vi "Run.vi"(7 "Team Index":i32, 8 "Column":i32, 9 "Row":i32, 10 "View":i32[](array[numeric]) caption="View (Team Index, -1: empty)", 11 "Test In":refnum<class "Swarm.lvclass">) -> (0 "Replicated":refnum<class "Square.lvclass">, 1 "Direction":T1, 2 "Action":T2, 3 "Square Out":refnum<class "Square.lvclass">)   [LabVIEW 2017, in "Swarm.lvclass"]
uses:
  Swarm.lvclass
  C:/Workspace/Endigit/SquareBattle/Square/Square.lvclass
  Square/Square.lvclass
  Type Defs/Action Enum.ctl
  Type Defs/Direction Enum.ctl
  Common/Position.ctl
  Swarm.lvclass/Swarm.ctl
  SubVIs/Read-Only Globals.vi
  SubVIs/Globals (private).vi
  Common/Common.lvlib
  Type Defs/SB Type Defs.lvlib
panel:
  # "NW\nN\nNE\nE\nSE\nS\nSW\nW"
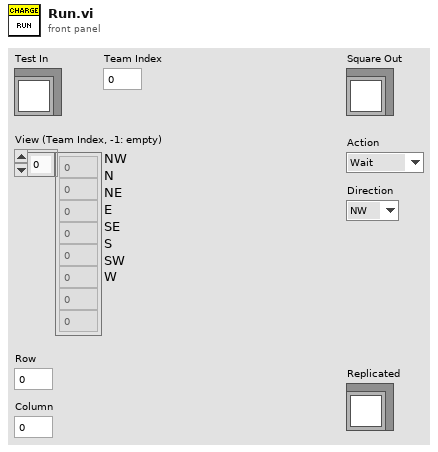
[diagram p1: front panel]
types:
  T1 = typedef "SB Type Defs.lvlib/Direction Enum.ctl" = enum16{"NW", "N", "NE", "E", "SE", "S", "SW", "W"}
  T2 = typedef "SB Type Defs.lvlib/Action Enum.ctl" = enum16{"Wait", "Move", "Attack", "Replicate"}
  T3 = typedef "Common.lvlib/Position.ctl" = cluster{"Column":i32, "Row":i32}
  T4 = typedef "Common.lvlib/Map DVR.ctl" = refnum<data-value>
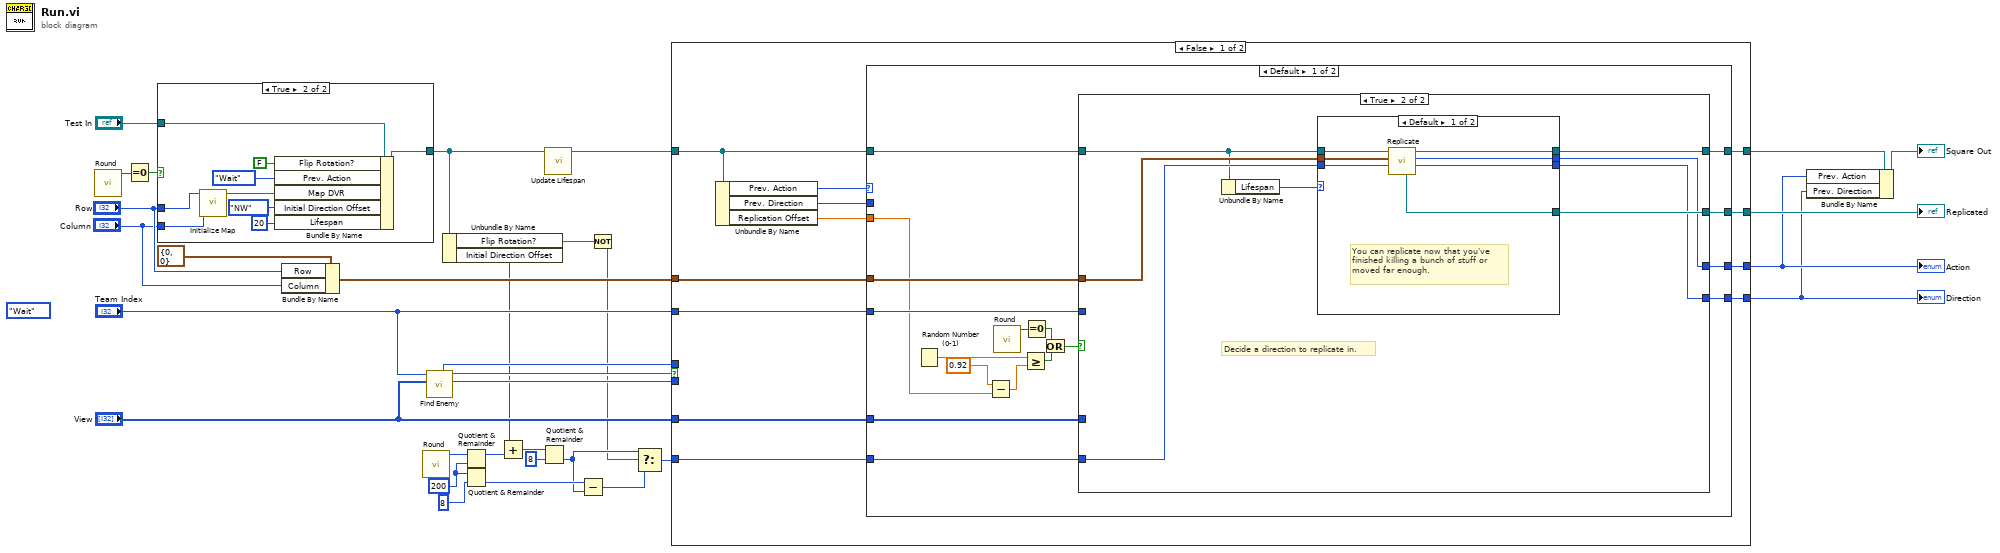
[diagram p0: block diagram]
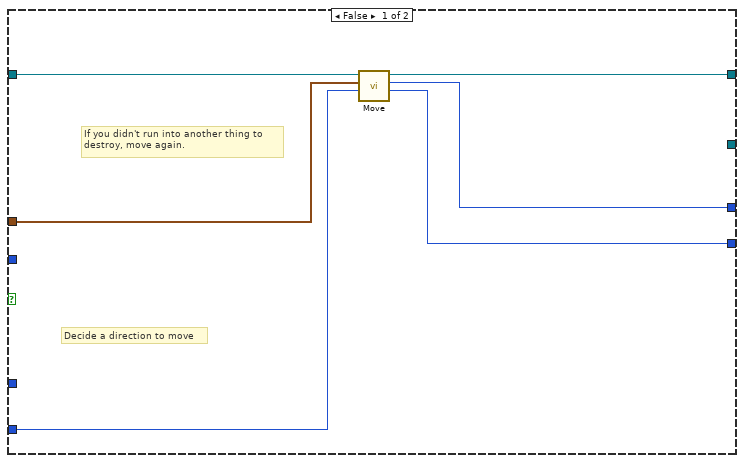
[diagram p3: hidden frame]
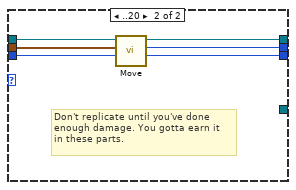
[diagram p4: hidden frame]
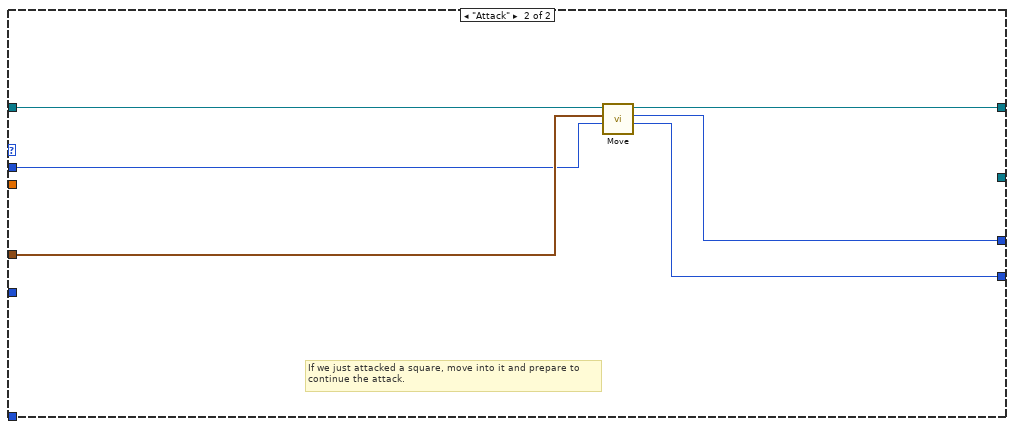
[diagram p5: hidden frame]
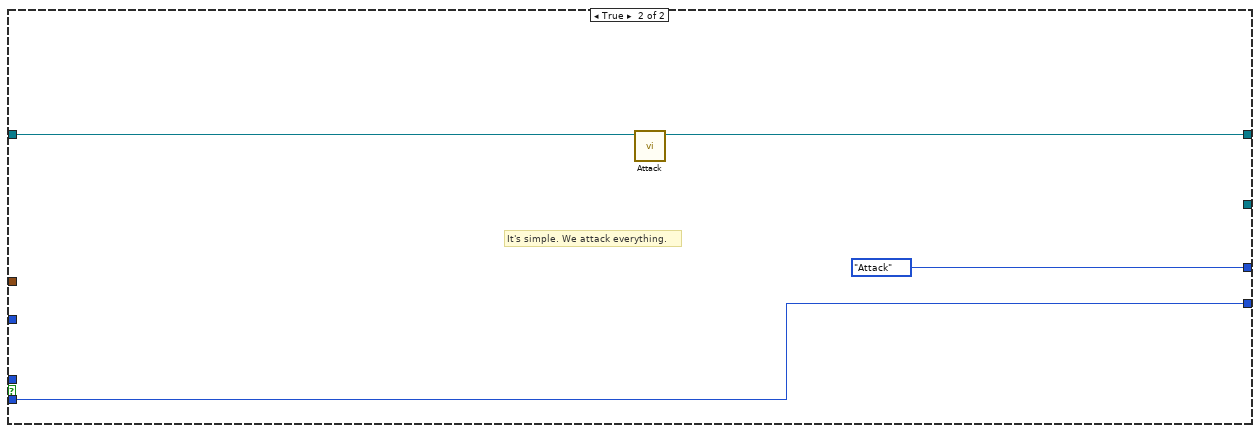
[diagram p6: hidden frame]
diagram:
  w8 = 200
  (unwired) Action_Enum."Wait" ("Action")
  n1 = call "Round.vi"() -> ("Round"=w27:i32)  [unwired: 11 in]
  n2 = Equal To 0?(x=w27) -> (x = 0?=w25:bool)
  n3 = case shown="True" w25 {
    tunnel: "Test In" -> [w33 w39]
    tunnel: [w33 w38] -> w9
    tunnel: "Row" -> [_ w42]
    tunnel: "Column" -> [_ w41]
    frame False {
    }
    frame True {
      n4 = call "Initialize Map.vi"("Column"=w41, "Row"=w42) -> ("Map DVR"=w40:T4)  [unwired: 9 in]
      n5 = Bundle By Name(cluster=w39, "Flip Rotation?"=FALSE, "Prev. Action"=Action_Enum."Wait", "Map DVR"=w40, "Initial Direction Offset"=Direction_Enum."NW", "Lifespan"=20) -> (w38:refnum<class "Swarm.lvclass">)
    }
  }
  n6 = Bundle By Name(cluster=T3 {"Column"=0, "Row"=0} ("Position in"), "Row"="Row", "Column"="Column") -> (w23:T3)
  n7 = call "Round.vi"() -> ("Round"=w19:i32)  [unwired: 11 in]
  n8 = call "Find Enemy.vi"("View"="View", "Team Index"="Team Index") -> ("Direction"=w31:T1, "Found Enemy?"=w32:bool, "Enemy"=w28:i32)  [unwired: 7 in]
  n9 = Unbundle By Name(w9) -> ("Flip Rotation?"=w2:bool, "Initial Direction Offset"=w12:T1)
  n10 = Quotient & Remainder(x=w19, y=w8) -> (x-y*floor(x/y)=w13:i32)  [unwired: 1 out]
  n11 = Quotient & Remainder(x=w8, y=8) -> (floor(x/y)=w6:i32)  [unwired: 1 out]
  n12 = Add(x=w12, y=w13) -> (x+y=w11:i32)
  n13 = Quotient & Remainder(x=w11, y=8) -> (floor(x/y)=w4:i32)  [unwired: 1 out]
  n14 = call-dynamic "Update Lifespan.vi"("Test in"=w9) -> ("Test out"=w10:refnum<class "Swarm.lvclass">)  [unwired: 9 in, 1 out]
  n15 = Subtract(x=w6, y=w4) -> (x-y=w5:i32)
  n16 = Not(x=w2) -> (.not. x?=w1:bool)
  n17 = Select(t=w4, s=w1, f=w5) -> (s? t:f=w3:i32)
  n18 = case shown="False" w32 {
    tunnel: w31 -> [_ w108]
    tunnel: "View" -> [w53 _]
    tunnel: "Team Index" -> [w54 _]
    tunnel: [w49 w108] -> w14
    tunnel: w28 -> [_ _]
    tunnel: [w50 Action_Enum."Attack" ("Action")] -> w15
    tunnel: [w52 w105] -> w16
    tunnel: w10 -> [w46 w106]
    tunnel: w23 -> [w51 _]
    tunnel: [w48 _] -> w20
    tunnel: w3 -> [w47 _]
    frame False {
      n19 = Unbundle By Name(w46) -> ("Prev. Action"=w45:T2, "Prev. Direction"=w44:T1, "Replication Offset"=w43:dbl)
      n20 = case shown="Default" w45 {
        tunnel: w54 -> [w70 _]
        tunnel: w53 -> [w69 _]
        tunnel: [w64 w104] -> w52
        tunnel: w51 -> [w63 w103]
        tunnel: [w62 w102] -> w50
        tunnel: [w61 w101] -> w49
        tunnel: [w60 _] -> w48
        tunnel: w47 -> [w59 _]
        tunnel: w46 -> [w58 w100]
        tunnel: w44 -> [_ w99]
        tunnel: w43 -> [w57 _]
        frame Default {
          n21 = Random Number (0-1)() -> (number: 0 to 1=w71:dbl)
          n22 = Subtract(x=0.92, y=w57) -> (x-y=w55:dbl)
          n23 = call "Round.vi"() -> ("Round"=w68:i32)  [unwired: 11 in]
          n24 = Greater Or Equal?(x=w71, y=w55) -> (x >= y?=w66:bool)
          n25 = Equal To 0?(x=w68) -> (x = 0?=w67:bool)
          n26 = Or(x=w67, y=w66) -> (x .or. y?=w65:bool)
          n27 = case shown="True" w65 {
            tunnel: w70 -> [_ _]
            tunnel: w69 -> [_ _]
            tunnel: [w76 w85] -> w64
            tunnel: w58 -> [w77 w79]
            tunnel: w63 -> [w75 w84]
            tunnel: [w73 w81] -> w62
            tunnel: [w72 w80] -> w61
            tunnel: [_ w82] -> w60
            tunnel: w59 -> [w74 w83]
            frame False {
              # "If you didn't run into another thing to\ndestroy, move again."
              # "Decide a direction to move"
              n28 = call-dynamic "Move.vi"("Direction Offset"=w74, "Current Position"=w75, "Test in"=w77) -> ("Direction"=w72:T1, "Action"=w73:T2, "Test out"=w76:refnum<class "Swarm.lvclass">)  [unwired: 5 in, 1 out]
            }
            frame True {
              # "Decide a direction to replicate in."
              n29 = Unbundle By Name(w79) -> ("Lifespan"=w78:i32)
              n30 = case shown="Default" w78 {
                tunnel: [w92 w95] -> w85
                tunnel: w84 -> [w91 w97]
                tunnel: w83 -> [w90 w96]
                tunnel: [w89 _] -> w82
                tunnel: [w88 w94] -> w81
                tunnel: [w87 w93] -> w80
                tunnel: w79 -> [w86 w98]
                frame Default {
                  # "You can replicate now that you've\nfinished killing a bunch of stuff or\nmoved far enough."
                  n31 = call-dynamic "Replicate.vi"("Direction Offset"=w90, "Current Position"=w91, "Test in"=w86) -> ("Direction"=w87:T1, "Action"=w88:T2, "Test out"=w92:refnum<class "Swarm.lvclass">, "Replicated"=w89:refnum<class "Swarm.lvclass">)  [unwired: 4 in, 1 out]
                }
                frame ..20 {
                  # "Don't replicate until you've done\nenough damage. You gotta earn it\nin these parts."
                  n32 = call-dynamic "Move.vi"("Direction Offset"=w96, "Current Position"=w97, "Test in"=w98) -> ("Direction"=w93:T1, "Action"=w94:T2, "Test out"=w95:refnum<class "Swarm.lvclass">)  [unwired: 5 in, 1 out]
                }
              }
            }
          }
        }
        frame "Attack" {
          # "If we just attacked a square, move into it and prepare to\ncontinue the attack."
          n33 = call-dynamic "Move.vi"("Direction Offset"=w99, "Current Position"=w103, "Test in"=w100) -> ("Direction"=w101:T1, "Action"=w102:T2, "Test out"=w104:refnum<class "Swarm.lvclass">)  [unwired: 5 in, 1 out]
        }
      }
    }
    frame True {
      # "It's simple. We attack everything."
      n34 = call-dynamic "Attack.vi"("Test in"=w106) -> ("Test out"=w105:refnum<class "Swarm.lvclass">)  [unwired: 9 in, 1 out]
    }
  }
  "Action" <- w15
  "Direction" <- w14
  "Replicated" <- w20
  n35 = Bundle By Name(cluster=w16, "Prev. Action"=w15, "Prev. Direction"=w14) -> (→"Square Out":refnum<class "Swarm.lvclass">)
